vi "Create Arbitrary Sequence [SEQ] Core.vi"(8 "error in (no error)":errorcluster, 9 "waveform handles array (empty)":i32[](array[numeric]), 10 "loop counts array (empty)":i32[](array[numeric]), 11 "IVI_Fgen in":refnum<class "IVI_Fgen.lvclass">) -> (0 "error out":errorcluster, 2 "sequence handle":i32, 3 "IVI_Fgen out":refnum<class "IVI_Fgen.lvclass">)   [LabVIEW 2013, in "IVI_Fgen.lvlib" / "IVI_Fgen.lvclass"]
doc: "An arbitrary sequence consists of multiple waveforms. For each waveform, you specify the number of times the function generator produces the waveform before proceeding to the next waveform. The number of times to repeat a specific waveform is called the loop count.\n \nThis VI creates an arbitrary sequence from an array of waveform handles and an array of corresponding loop counts. The VI returns a handle that identifies the sequence. You pass this handle to the IviFgen Configure Arbitrary Sequence [SEQ] VI to specify what arbitrary sequence you want the function generator to produce.\n\nNotes:\n\n(1) This VI is part of the IviFgenArbSeq [SEQ] extension group."
uses:
  IVI_Fgen.lvclass
  IVI_Fgen.lvclass/IVI_Fgen.ctl
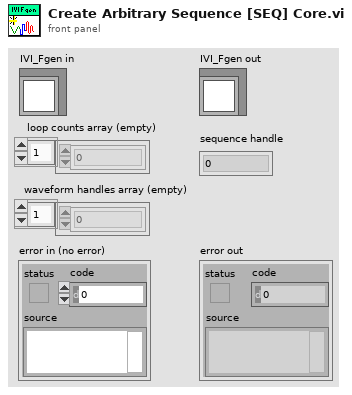
[diagram p1: front panel]
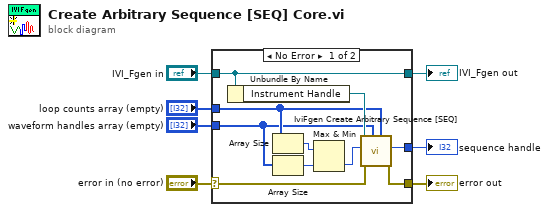
[diagram p0: block diagram]
diagram:
  n1 = case shown="No Error" "error in (no error)" {
    selector: "error in (no error)" -> [w15 w19]
    tunnel: [w14 w19] -> w6
    tunnel: [w17 w18] -> w4
    tunnel: "IVI_Fgen in" -> [w17 w18]
    tunnel: [w13 _] -> w3
    tunnel: "loop counts array (empty)" -> [w12 _]
    tunnel: "waveform handles array (empty)" -> [w11 _]
    frame No Error {
      n2 = Unbundle By Name(w17) -> ("Instrument Handle"=w16:refnum<k15>)
      n3 = Array Size(array=w12) -> (size(s)=w10:i32)
      n4 = Array Size(array=w11) -> (size(s)=w9:i32)
      n5 = Max & Min(x=w10, y=w9) -> (min(x,y)=w8:i32)  [unwired: 1 out]
      n6 = call <vilib>:"IviFgen Create Arbitrary Sequence [SEQ].vi"("loop counts array (empty)"=w12, "waveform handles array (empty)"=w11, "error in (no error)"=w15, "sequence length (1)"=w8, "instrument handle"=w16) -> ("error out"=w14:errorcluster, "sequence handle"=w13:i32)  [unwired: 4 in, 1 out]
    }
    frame Error {
    }
  }
  "error out" <- w6
  "IVI_Fgen out" <- w4
  "sequence handle" <- w3
